vi "Write Path.vi"(8 "error in (no error)":errorcluster, 10 "Path":path, 11 "Datalogger Path Set in":refnum<class "Datalogger Path Set Message.lvclass">) -> (0 "error out":errorcluster, 3 "Datalogger Path Set out":refnum<class "Datalogger Path Set Message.lvclass">)   [LabVIEW 2018, in "Datalogger Path Set Message.lvclass"]
uses:
  Datalogger Path Set Message.lvclass
  Datalogger Path Set Message.lvclass/Datalogger Path Set Message.ctl
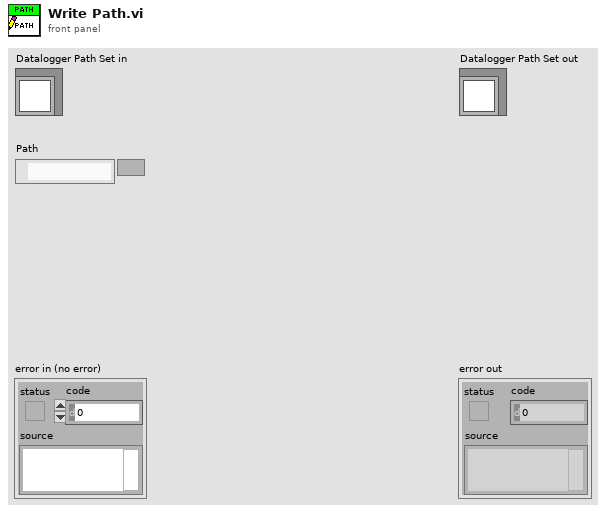
[diagram p1: front panel]
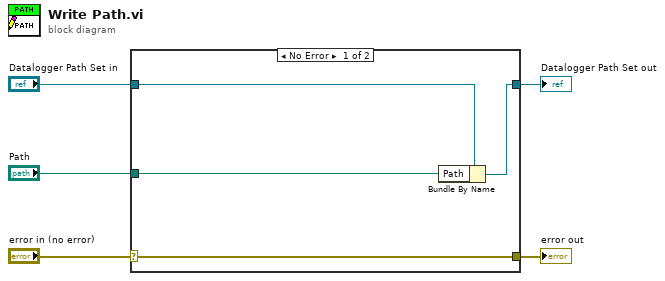
[diagram p0: block diagram]
diagram:
  n1 = case shown="No Error" "error in (no error)" {
    selector: "error in (no error)" -> [w9 w10]
    tunnel: [w9 w10] -> w4
    tunnel: [w7 w11] -> w2
    tunnel: "Datalogger Path Set in" -> [w8 w11]
    tunnel: "Path" -> [w6 _]
    frame No Error {
      n2 = Bundle By Name(cluster=w8, "Path"=w6) -> (w7:refnum<class "Datalogger Path Set Message.lvclass">)
    }
    frame Error {
    }
  }
  "error out" <- w4
  "Datalogger Path Set out" <- w2
